vi "Build_Write Single Coil.vi"(8 "error in (no error)":errorcluster, 9 "value":bool, 10 "address":u16) -> (0 "error out":errorcluster, 3 "MB_PDU":T1={"Function Code"=1, "Data"=[], "RTU_DataBytes"=0})   [LabVIEW 2021, in "MB Master.lvlib"]
doc: "Builds PDU for Write Single Coil (function code 5)."
uses:
  <vilib>/Plasmionique/MB Master/MB Master.lvlib
  <vilib>/Plasmionique/MB Master/MB_PDU/MB_PDU_Cluster.ctl
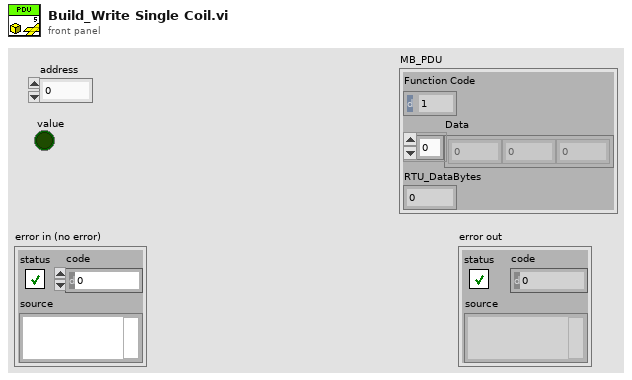
[diagram p1: front panel]
types:
  T1 = typedef "MB Master.lvlib/MB_PDU_Cluster.ctl" = cluster{"Function Code":u8, "Data":u8[], "RTU_DataBytes":i32}
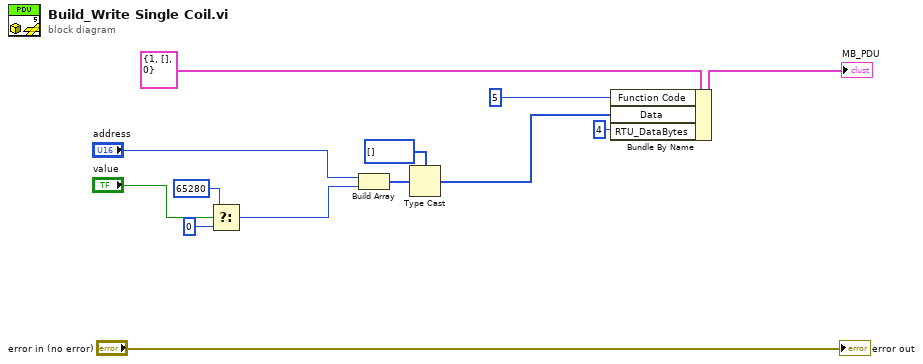
[diagram p0: block diagram]
diagram:
  n1 = Select(t=u16 65280, s="value", f=u16 0) -> (s? t:f=w2:u16)
  n2 = Build Array("address", w2) -> (w13:u16[])
  n3 = Type Cast(type=u8[] [], x=w13) -> (*(type *) &x=w8:u8[])
  n4 = Bundle By Name(cluster=T1 {"Function Code"=1, "Data"=[], "RTU_DataBytes"=0} ("Modbus Serial New.lvlib:MB_PDU.lvclass"), "Function Code"=u8 5, "Data"=w8, "RTU_DataBytes"=4 ("NumBytes")) -> (→"MB_PDU":T1)
  "error out" <- "error in (no error)"
